vi "YOLOv5_OpenVINO_IR.vi"() -> ()   [LabVIEW 2018]
doc: "YOLOv5_OpenVINO_IR: This example is an object detection example of the YOLOv5 algorithm, which can perform object detection on real-time images captured by cameras. IR is OpenVINO's proprietary optimized format model."
uses:
  vi.lib/VIRobotics/ModelZoo/Object_Detection/yolov5_openvino/InitialModel_yolov5_OpenVINO_IR.vi
  vi.lib/VIRobotics/opencv_yiku/Cap/Cap.lvclass
  vi.lib/VIRobotics/ModelZoo/Object_Detection/yolov5_openvino/yolov5_openvino.lvclass
  vi.lib/VIRobotics/opencv_yiku/Mat/Mat_8U/Mat_8U.lvclass
panel:
  in  "device_name":string(combo)="CPU"
  in  "config":T1={"confThreshold"=0.3, "nms_threshold"=0.5, "fontScale"=0.5}
  in  "bin_fle":path=path "C:/ProgramData/VIRobotics/ModelZoo/Object_Detection/yolov5/IR_model/yolov5s.bin"
  out "每帧耗时(s)":dbl
  in  "class_names_file":path=path "C:/ProgramData/VIRobotics/ModelZoo/Object_Detection/coco.names"
  in  "xml_file":path=path "C:/ProgramData/VIRobotics/ModelZoo/Object_Detection/yolov5/IR_model/yolov5s.xml"
  in  "stop":bool
  out "picture":picture
  # "Overview: Demonstrates how to use OpenVINO to load the the IR model of yolov5 for real-time object detection.\nRequirements: Windows.\nMake sure your computer has a camera。\nInstructions: \n1.Select the device_name to use.（If your computer has Intel GPU, you can select GPU in the \"type\" control before running the VI to achieve faster inference).\n2.Run the VI.\nIf you want to load the model you trained, follow the following steps:\n1.Select the device_name to use. \n2.Specify the xml_file、bin_file and class_names_file.\n3.Run the VI."
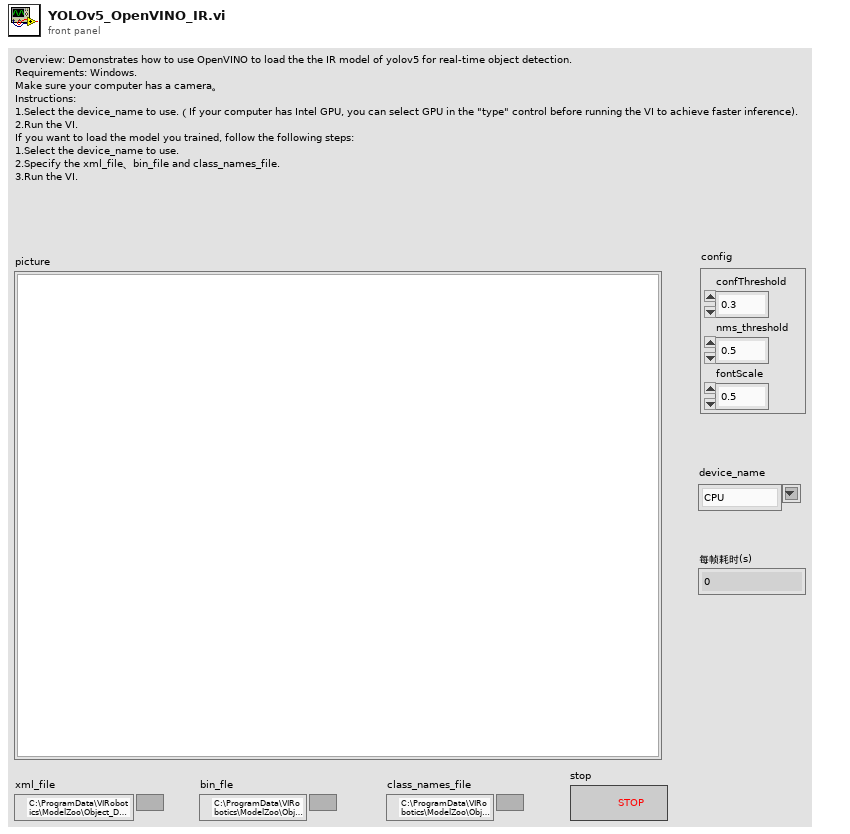
[diagram p1: front panel]
types:
  T1 = cluster{"confThreshold":sgl, "nms_threshold":sgl, "fontScale":dbl}
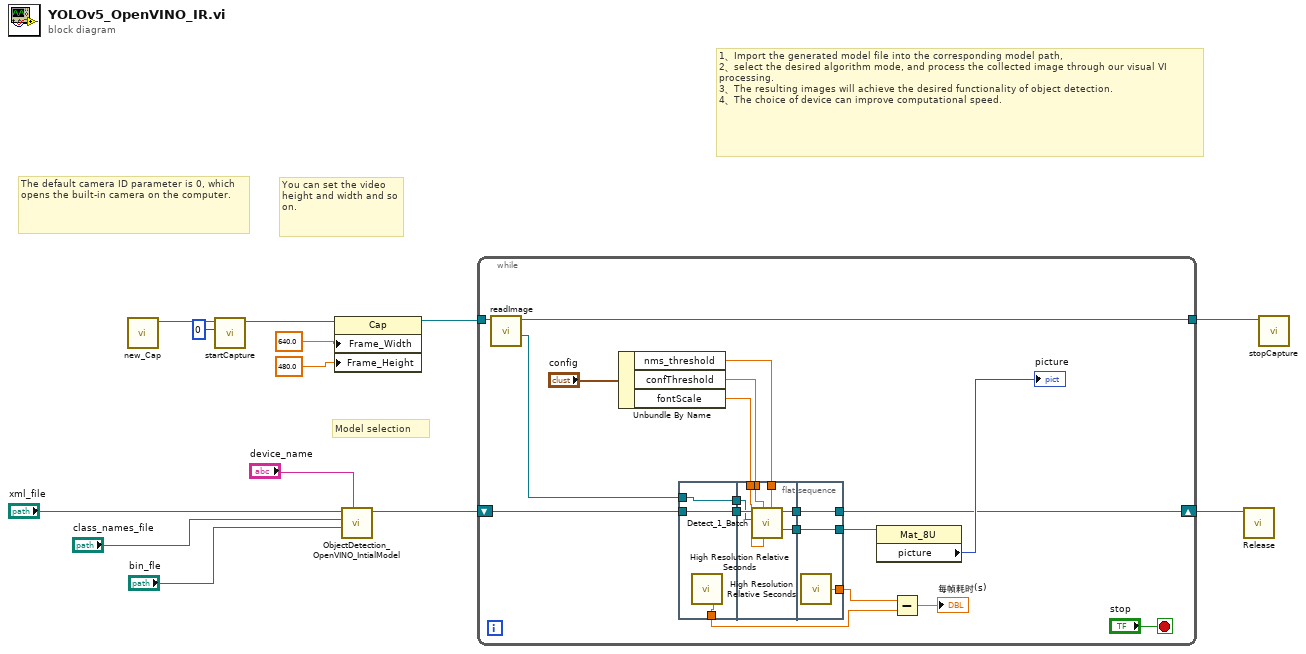
[diagram p0: block diagram]
diagram:
  # "1、Import the generated model file into the corresponding model path, \n2、select the desired algorithm mode, and process the collected image through our visual VI processing. \n3、The resulting images will achieve the desired functionality of object detection. \n4、The choice of device can improve computational speed."
  # "Model selection"
  # "You can set the video height and width and so on."
  # "The default camera ID parameter is 0, which opens the built-in camera on the computer."
  n1 = call "new_Cap.vi"() -> ("Cap out"=w7:refnum<class "Cap.lvclass">)  [unwired: 10 in, 1 out]
  n2 = call "startCapture.vi"("cameraID"=0, "Cap in"=w7) -> ("Cap out"=w4:refnum<class "Cap.lvclass">)  [unwired: 8 in, 1 out]
  n3 = property class="Cap"(reference=w4, "Frame_Width"=640.0, "Frame_Height"=480.0) -> (reference out=w2:refnum<class "Cap.lvclass">)  [unwired: 1 in, 1 out]
  n4 = call-poly "ObjectDetection_OpenVINO_IntialModel.vi"("device_name"="device_name", "bin_fle"="bin_fle", "class_names_path"="class_names_file", "xml path"="xml_file") -> ("yolov5_openvino out"=w11:refnum<class "yolov5_openvino.lvclass">)  [unwired: 6 in, 1 out]
  n5 = while {
    tunnel: w2 -> [w31]
    shift-right: [w27] -> w12
    shift-left: w11 -> [w32]
    tunnel: [w26] -> w13
    stop <- "stop" stop-if-true
    n6 = call "readImage.vi"("Cap in"=w31) -> ("Mat out"=w19:refnum<class "Mat_8U.lvclass">, "Cap out"=w26:refnum<class "Cap.lvclass">)  [unwired: 8 in, 1 out]
    n7 = Unbundle By Name("config") -> ("nms_threshold"=w16:sgl, "confThreshold"=w15:sgl, "fontScale"=w14:dbl)
    n8 = flat-sequence {
      tunnel: w32 -> [w35]
      tunnel: [w35] -> w25
      tunnel: [w34] -> w21
      tunnel: w19 -> [w33]
      tunnel: [w33] -> w18
      tunnel: w25 -> [w42]
      tunnel: [w41] -> w24
      tunnel: [w40] -> w23
      tunnel: w18 -> [w39]
      tunnel: w16 -> [w38]
      tunnel: w15 -> [w37]
      tunnel: w14 -> [w36]
      tunnel: [w44] -> w27
      tunnel: [w45] -> w30
      tunnel: w24 -> [w45]
      tunnel: w23 -> [w44]
      tunnel: [w43] -> w22
      frame #0 {
        n9 = call <vilib>:"High Resolution Relative Seconds.vi"() -> ("relative seconds"=w34:dbl)
      }
      frame #1 {
        n10 = call-dynamic "Detect_1_Batch.vi"("nms_threshold"=w38, "fontScale"=w36, "confThreshold"=w37, "image"=w39, "yolov5_openvino in"=w42) -> ("img out"=w41:refnum<class "Mat_8U.lvclass">, "yolov5_openvino out"=w40:refnum<class "yolov5_openvino.lvclass">)  [unwired: 3 in, 2 out]
      }
      frame #2 {
        n11 = call <vilib>:"High Resolution Relative Seconds.vi"() -> ("relative seconds"=w43:dbl)
      }
    }
    n12 = property class="Mat_8U"(reference=w30) -> ("picture"=→"picture":picture)  [unwired: 1 in, 2 out]
    n13 = Subtract(x=w22, y=w21) -> (x-y=→"每帧耗时(s)":dbl)
  }
  n14 = call-dynamic "Release.vi"("yolov5_openvino in"=w12) -> ()  [unwired: 9 in, 2 out]
  n15 = call "stopCapture.vi"("Cap in"=w13) -> ()  [unwired: 10 in, 1 out]
